vi "SigProc_subVI CDFNormal.vi"(10 "half-width":i32) -> (2 "CDF Normal":dbl[](array[numeric]))   [LabVIEW 2018, in "Sig2MS.lvclass"]
uses:
  Sig2MS.lvclass
  <vilib>/gmath/statdist.llb/Normal CDF.vi
  <vilib>/gmath/NI_Gmath.lvlib
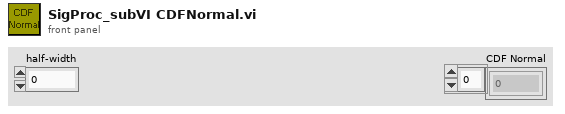
[diagram p1: front panel]
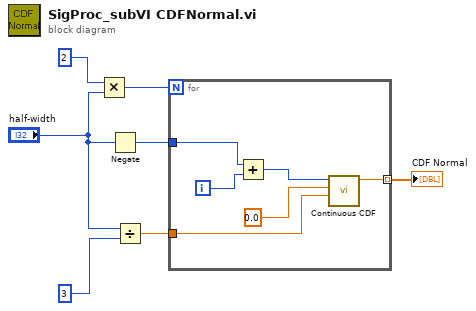
[diagram p0: block diagram]
diagram:
  n1 = Multiply(x=2 ("y"), y="half-width") -> (x*y=w1:i32)
  n2 = Negate(x="half-width") -> (-x=w6:i32)
  n3 = Divide(x="half-width", y=3) -> (x/y=w3:dbl)
  n4 = for {
    N: w1 -> [_]
    tunnel: w6 -> [w12]
    tunnel: w3 -> [w9]
    tunnel: [w8] -> w2 mode=indexing
    i -> [w13]
    n5 = Add(x=w12, y=w13) -> (x+y=w10:i32)
    n6 = call-poly <vilib>:"Continuous CDF.vi"("std"=w9, "mean"=0.0, "x"=w10) -> ("cdf(x)"=w8:dbl)  [unwired: 7 in, 1 out]
  }
  "CDF Normal" <- w2
